vi "Check Credential.vi"(8 "error in (no error)":errorcluster, 10 "Credential":T1, 11 "Access in":refnum<class "Access.lvclass">) -> (0 "error out":errorcluster, 2 "Match?":bool, 3 "Access out":refnum<class "Access.lvclass">)   [LabVIEW 2021, in "Database.lvlib" / "Access.lvclass"]
uses:
  Access.lvclass
  DB/Credential.ctl
  Access.lvclass/Access.ctl
  <vilib>/addons/database/NI_Database_API.lvlib
  Database.lvlib
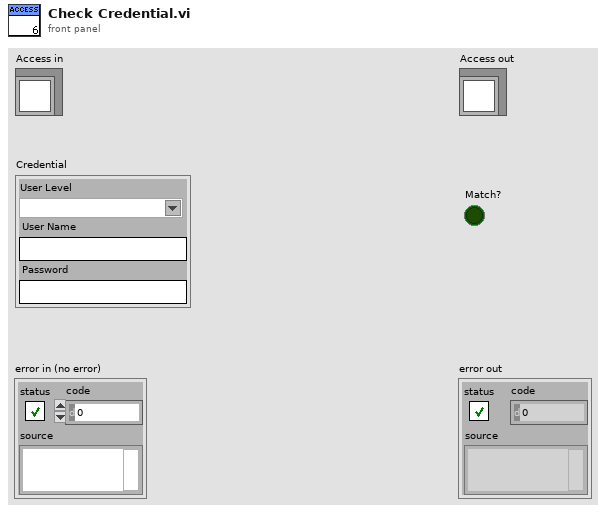
[diagram p1: front panel]
types:
  T1 = typedef "Database.lvlib/Credential.ctl" = cluster{"User Level":string, "User Name":string, "Password":string}
  T2 = typedef "Database.lvlib/DB.lvclass/Table_info.ctl" = cluster{"Authentication":string, "Instr_Configuration":string, "Recipe":string, "Test_data":string}
  T3 = typedef "NI_Database_API.lvlib/Conn ObjectReference.ctl" = refnum<k1>
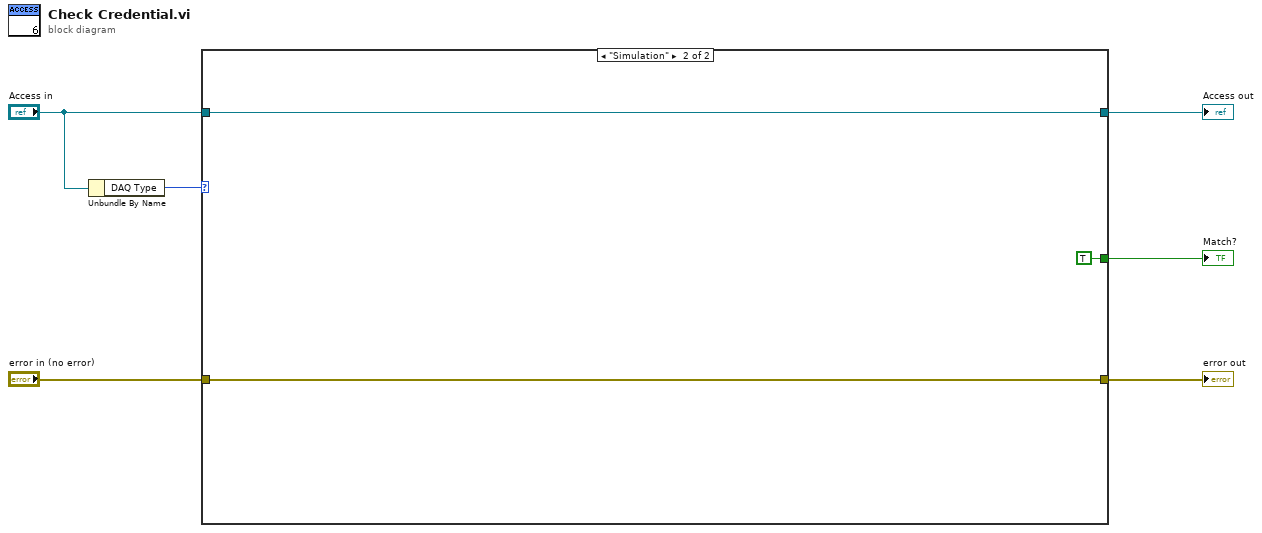
[diagram p0: block diagram]
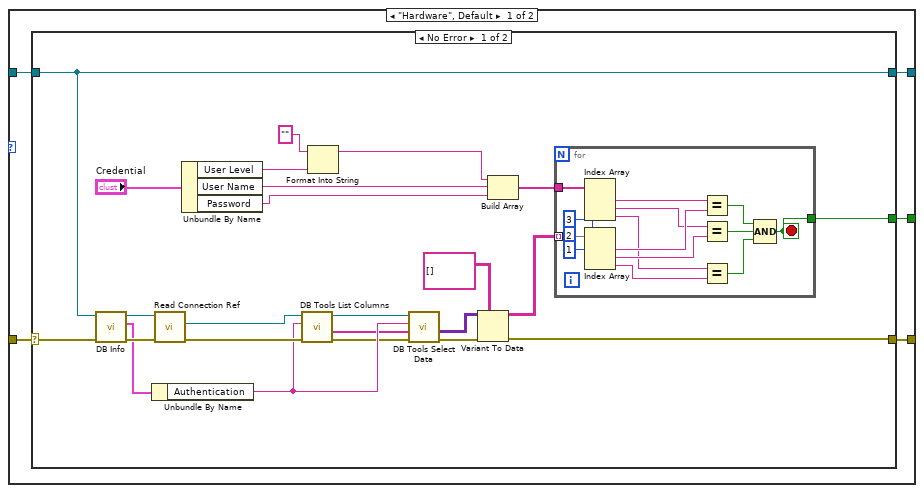
[diagram p2: hidden frame]
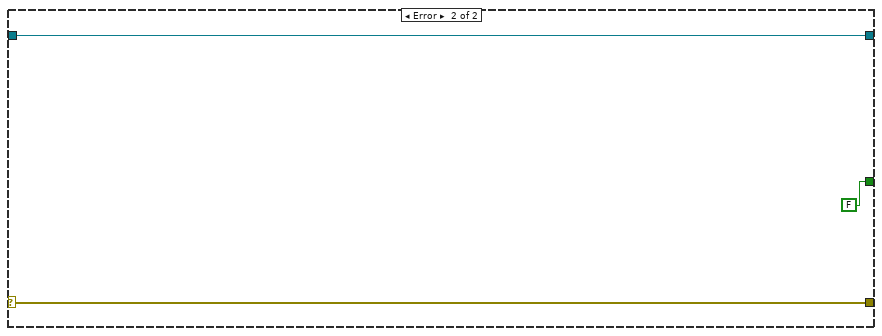
[diagram p3: hidden frame]
diagram:
  n1 = Unbundle By Name("Access in") -> ("DAQ Type"=w1:enum16{"Hardware", "Simulation"})
  n2 = case shown="\"Simulation\"" w1 {
    tunnel: "error in (no error)" -> [w11 w55]
    tunnel: [w10 w56] -> w5
    tunnel: [w9 w55] -> w4
    tunnel: [w8 TRUE] -> w3
    tunnel: "Access in" -> [w7 w56]
    frame "Hardware", Default {
      n3 = case shown="No Error" w11 {
        selector: w11 -> [w35 w52]
        tunnel: w7 -> [w33 w53]
        tunnel: [w33 w53] -> w10
        tunnel: [w21 w52] -> w9
        tunnel: [w12 FALSE] -> w8
        frame No Error {
          n4 = call-dynamic "DB Info.vi"("error in (no error)"=w35, "Access in"=w33) -> ("error out"=w34:errorcluster, "Table_info"=w31:T2, "Access out"=w32:refnum<class "Access.lvclass">)  [unwired: 6 in, 1 out]
          n5 = Unbundle By Name(w31) -> ("Authentication"=w28:string)
          n6 = call-dynamic "Read Connection Ref.vi"("error in (no error)"=w34, "Access in"=w32) -> ("error out"=w30:errorcluster, "connection reference"=w29:T3)  [unwired: 7 in, 1 out]
          n7 = Unbundle By Name("Credential") -> ("User Level"=w19:string, "User Name"=w15:string, "Password"=w14:string)
          n8 = call <vilib>:"DB Tools List Columns.vi"("error in (no error)"=w30, "table"=w28, "connection reference"=w29) -> ("error out"=w26:errorcluster, "columns"=w27:string[], "connection reference out"=w25:T3)  [unwired: 1 in, 1 out]
          n9 = Format Into String(initial string="", w19) -> (resulting string=w16:string)  [unwired: 2 in, 1 out]
          n10 = call <vilib>:"DB Tools Select Data.vi"("error in (no error)"=w26, "columns"=w27, "table"=w28, "connection reference"=w25) -> ("error out"=w24:errorcluster, "data"=w23:variant[][])  [unwired: 2 in, 1 out]
          n11 = Variant To Data(error in=w24, type=string[][] [], Variant=w23) -> (data=w17:string[][], error out=w21:errorcluster)
          n12 = Build Array(w16, w15, w14) -> (w13:string[])
          n13 = for {
            tunnel: w17 -> [w50] mode=indexing
            tunnel: w13 -> [w49]
            tunnel: [w39] -> w12
            stop <- w39 stop-if-true
            n14 = Index Array(array=w49) -> (element #1=w48:string, element #2=w46:string, element #3=w44:string)  [unwired: 3 in]
            n15 = Index Array(array=w50, index #1=1 ("index"), index #2=2 ("index"), index #3=3 ("index")) -> (element #1=w47:string, element #2=w45:string, element #3=w43:string)
            n16 = Equal?(x=w48, y=w47) -> (x = y?=w42:bool)
            n17 = Equal?(x=w46, y=w45) -> (x = y?=w41:bool)
            n18 = Equal?(x=w44, y=w43) -> (x = y?=w40:bool)
            n19 = Compound Arithmetic op=AND(w42, w41, w40) -> (w39:bool)
          }
        }
        frame Error {
        }
      }
    }
    frame "Simulation" {
    }
  }
  "error out" <- w4
  "Access out" <- w5
  "Match?" <- w3
